vi "开关电磁阀.vi"() -> ()   [LabVIEW 2013]
panel:
  in  "开关电磁阀":bool
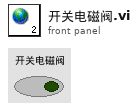
[diagram p1: front panel]
diagram:
